vi "Get-safe.vi"(8 "error in (no error)":errorcluster, 11 "Motor-Xaxis in":refnum<class "Motor-Xaxis.lvclass">) -> (0 "error out":errorcluster, 1 "Safe?":bool, 3 "Motor-Xaxis out":refnum<class "Motor-Xaxis.lvclass">)   [LabVIEW 2013, in "PowderDeposition.lvlib" / "Motor-Xaxis.lvclass"]
uses:
  Motor-Xaxis.lvclass
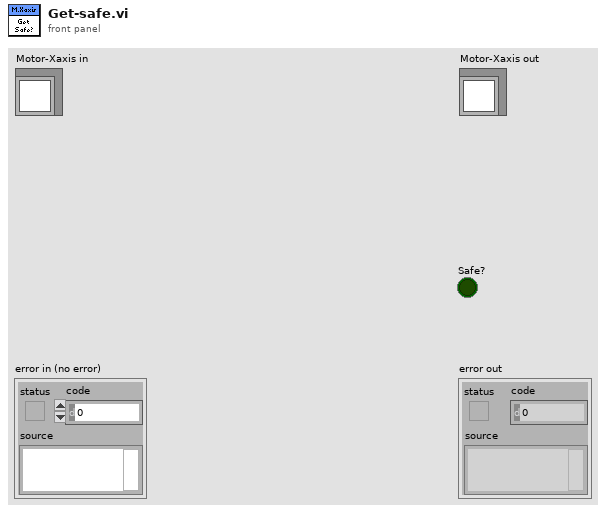
[diagram p1: front panel]
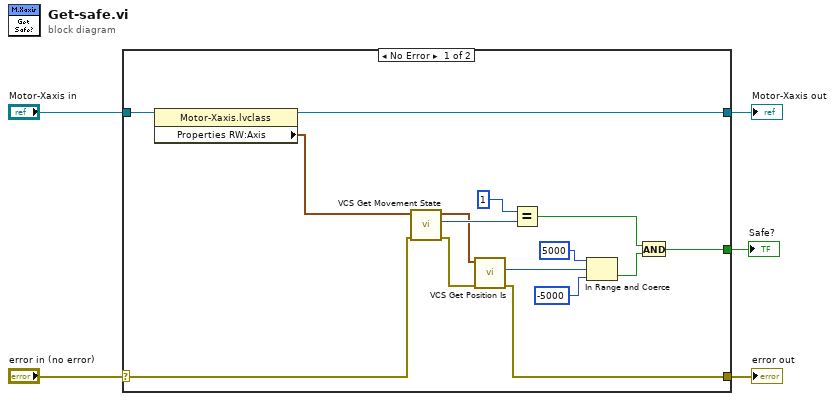
[diagram p0: block diagram]
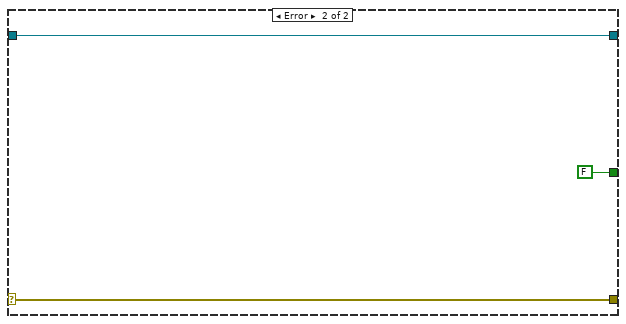
[diagram p2: hidden frame]
diagram:
  n1 = case shown="No Error" "error in (no error)" {
    selector: "error in (no error)" -> [w19 w23]
    tunnel: [w18 w23] -> w4
    tunnel: [w16 w22] -> w2
    tunnel: "Motor-Xaxis in" -> [w17 w22]
    tunnel: [w8 FALSE] -> w1
    frame No Error {
      n2 = property class="Motor-Xaxis.lvclass"(reference=w17) -> (reference out=w16:refnum<class "Motor-Xaxis.lvclass">, "Properties RW:Axis"=w7:cluster{"keyHandle":u32, "nodeID":u16})  [unwired: 1 in, 1 out]
      n3 = call <instrlib>:"VCS Get Movement State.vi"("error in (no error)"=w19, "axis in"=w7) -> ("error out"=w20:errorcluster, "targetReached"=w15:i32, "axis out"=w6:cluster{"keyHandle":u32, "nodeId":u16})  [unwired: 7 in]
      n4 = call <instrlib>:"VCS Get Position Is.vi"("error in (no error)"=w20, "axis in"=w6) -> ("error out"=w18:errorcluster, "positionIs"=w13:i32)  [unwired: 7 in, 1 out]
      n5 = Equal?(x=1, y=w15) -> (x = y?=w10:bool)
      n6 = In Range and Coerce(upper limit=5000, x=w13, lower limit=-5000) -> (In Range?=w9:bool)  [unwired: 1 out]
      n7 = And(x=w10, y=w9) -> (x .and. y?=w8:bool)
    }
    frame Error {
    }
  }
  "error out" <- w4
  "Motor-Xaxis out" <- w2
  "Safe?" <- w1
